vi "MDAQ_OldRawDataParser.vi"(8 "error in":errorcluster, 11 "Raw Data In":string[](array[string])) -> (0 "error out":errorcluster, 2 "Run Data Cluster":T1 {"Temperature B" scale=0.0..100.0; "Temperature A" scale=0.0..100.0}, 3 "SetPoints array":i32[](array[numeric]))   [LabVIEW 2021]
uses:
  DAT_Cluster.ctl
  68631d53-2441-47b5-8ba3-829a2f4a7f07.vi
  c980f971-6339-4fa8-b591-5bab5b2ab94e.vi
  <vilib>/Comparison/Less/Less Functor/Less Functor.lvclass
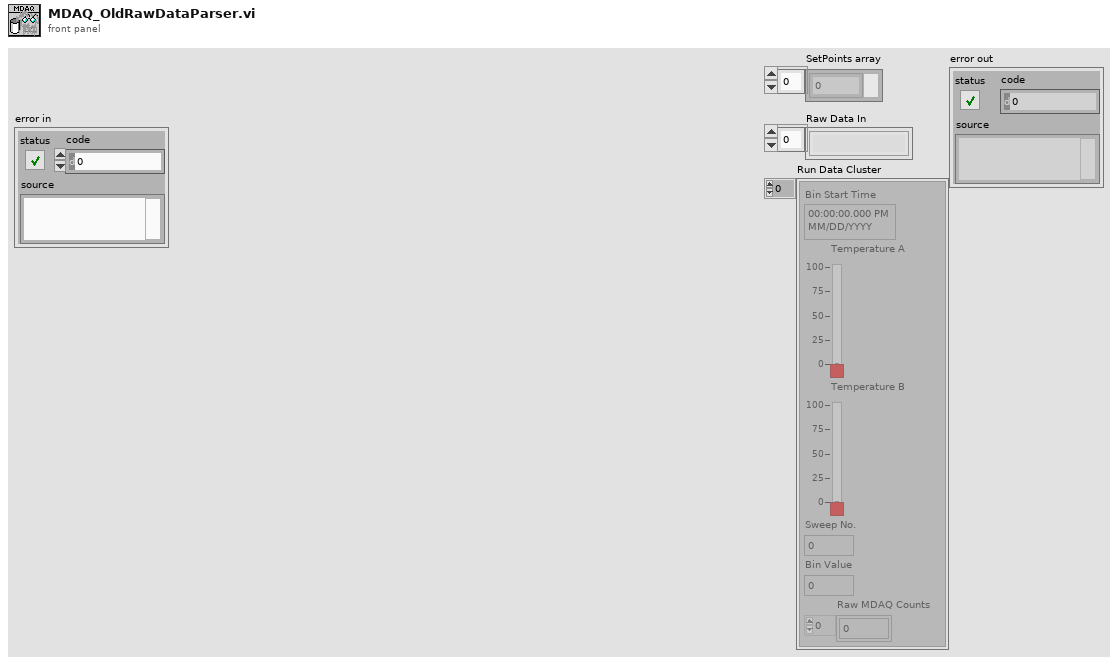
[diagram p1: front panel]
types:
  T1 = typedef "DAT_Cluster.ctl" = cluster{"Bin Start Time":timestamp, "Temperature A":dbl, "Temperature B":dbl, "Sweep No.":i32, "Bin Value":i32, "Raw MDAQ Counts":i32[]}[]
  T2 = cluster{"Bin Start Time":timestamp, "Temperature A":dbl, "Temperature B":dbl, "Sweep No.":i32, "Bin Value":i32, "Raw MDAQ Counts":i32[]}
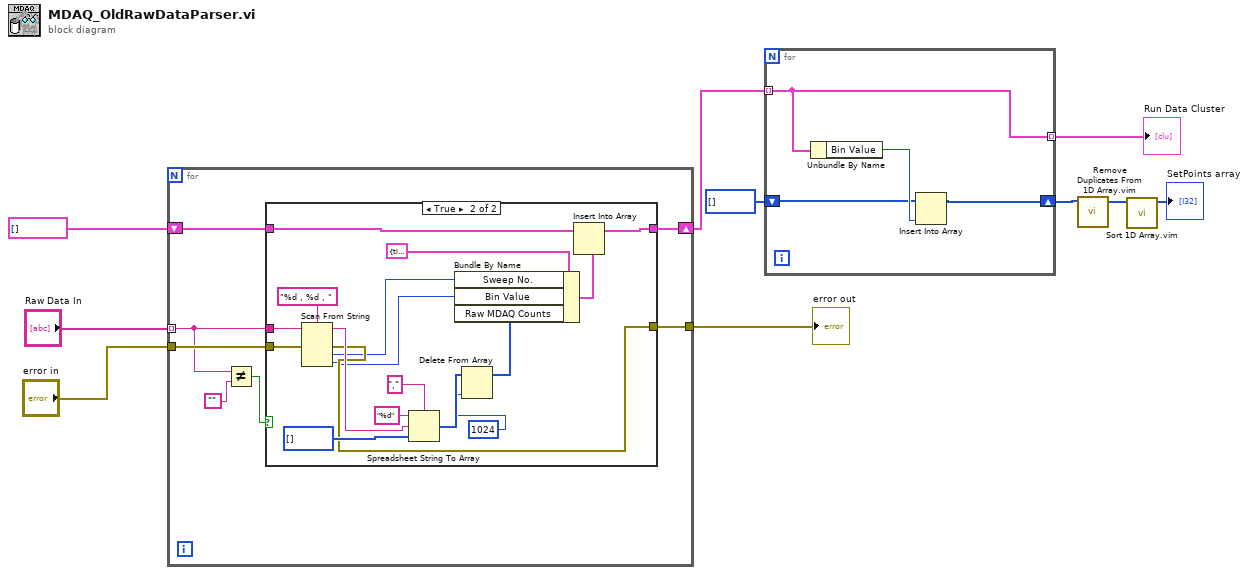
[diagram p0: block diagram]
diagram:
  n1 = for {
    tunnel: "Raw Data In" -> [w13] mode=indexing
    tunnel: "error in" -> [w17]
    shift-right: [w15] -> w6
    shift-left: T1 [] ("Run Data Cluster") -> [w16]
    tunnel: [w14] -> w7
    n2 = Not Equal?(x=w13, y="") -> (x != y?=w11:bool)
    n3 = case shown="True" w11 {
      tunnel: w13 -> [_ w36]
      tunnel: w17 -> [w18 w35]
      tunnel: w16 -> [w19 w33]
      tunnel: [w19 w30] -> w15
      tunnel: [w18 w25] -> w14
      frame False {
      }
      frame True {
        n4 = Scan From String(format string="%d , %d , ", input string=w36, error in=w35) -> (remaining string=w28:string, error out=w25:errorcluster, output 1=w24:i32, output 2=w23:i32)  [unwired: 3 in, 1 out]
        n5 = Spreadsheet String To Array(delimiter (Tab)=",", format string="%d", spreadsheet string=w28, array type (2D Dbl)=i32[] [] ("Raw MDAQ Counts")) -> (array=w22:i32[])
        n6 = Delete From Array(array=w22, index=1024) -> (array with subset deleted=w20:i32[])  [unwired: 1 in, 1 out]
        n7 = Bundle By Name(cluster=T2 {"Bin Start Time"=timestamp(0 s since 1904-01-01), "Temperature A"=0.0, "Temperature B"=0.0, "Sweep No."=0, "Bin Value"=0, "Raw MDAQ Counts"=[]} ("new element/subarray"), "Sweep No."=w24, "Bin Value"=w23, "Raw MDAQ Counts"=w20) -> (w31:T2)
        n8 = Insert Into Array(array=w33, new element=w31) -> (w30:T1)  [unwired: 1 in]
      }
    }
  }
  "error out" <- w7
  n9 = for {
    tunnel: w6 -> [w40] mode=indexing
    tunnel: [w40] -> w5 mode=indexing
    shift-right: [w38] -> w3
    shift-left: i32[] [] -> [w37]
    n10 = Unbundle By Name(w40) -> ("Bin Value"=w39:i32)
    n11 = Insert Into Array(array=w37, new element=w39) -> (w38:i32[])  [unwired: 1 in]
  }
  "Run Data Cluster" <- w5
  n12 = call "Remove Duplicates From 1D Array.vim"("array"=w3) -> ("array with duplicates removed"=w2:i32[])  [unwired: 10 in]
  n13 = call "Sort 1D Array.vim"("unsorted array"=w2) -> ("sorted array"=→"SetPoints array":i32[])  [unwired: 10 in]
